vi "GEA3 Read Write Example.vi"() -> ()   [LabVIEW 2020]
uses:
  type defs/ERD Write Data In.ctl
  type defs/Data Type.ctl
  type defs/ERD Read Data Out.ctl
  type defs/Source_Destination.ctl
  type defs/ERD Read Data In.ctl
  library/GEA2_Toolkit.lvlib
panel:
  out "String":string
  in  "Personality":string(combo)
  out "ERD Read Data Out":T1 {"ERD Number" format="%.0x"}
  in  "ERD Write Data In":T2 {"ERD Number" format="%.0x"}
  out "Raw Data Out":string
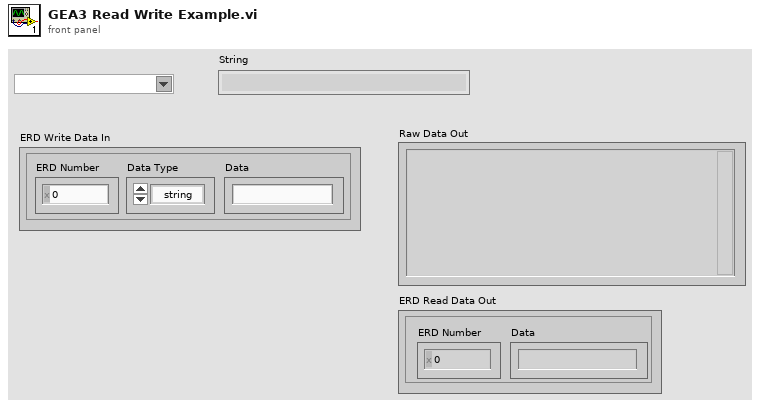
[diagram p1: front panel]
types:
  T1 = typedef "GEA2_Toolkit.lvlib/ERD Read Data Out.ctl" = cluster{"ERD Number":u16, "Data":string}
  T2 = typedef "GEA2_Toolkit.lvlib/ERD Write Data In.ctl" = cluster{"ERD Number":u16, "Data Type":T3, "Data":string}
  T3 = typedef "GEA2_Toolkit.lvlib/Data Type.ctl" = enum16{"string", "boolean", "uint8_t", "uint16_t", "uint32_t", "uint64_t", "int8_t", "int16_t", "int32_t", "int64_t"}
  T4 = typedef "GEA2_Toolkit.lvlib/ERD Read Data In.ctl" = cluster{"ERD Number":u16, "Data Type":T3}
  T5 = typedef "GEA2_Toolkit.lvlib/Source_Destination.ctl" = cluster{"Source":u8, "Destination":u8}
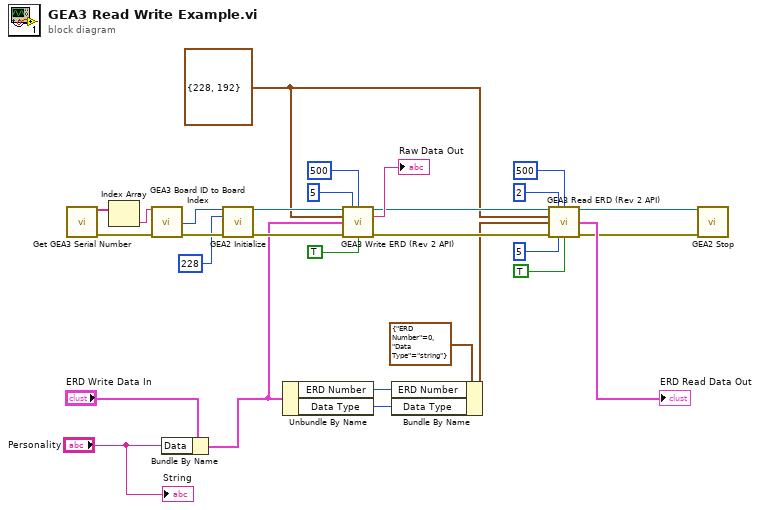
[diagram p0: block diagram]
diagram:
  w4 = T5 {"Source"=228, "Destination"=192} ("GEA Inputs")
  n1 = call "Get GEA3 Serial Number.vi"() -> ("GEA3 Serial Numbers"=w26:string[], "Error Out"=w27:errorcluster)  [unwired: 14 in]
  n2 = Index Array(array=w26) -> (element=w25:string)  [unwired: 1 in]
  n3 = call "GEA3 Board ID to Board Index.vi"("GEA3 Serial Number"=w25, "Error In"=w27) -> ("Board Index"=w28:i32, "Error Out"=w29:errorcluster)  [unwired: 9 in, 3 out]
  n4 = Bundle By Name(cluster="ERD Write Data In", "Data"="Personality") -> (w2:T2)
  n5 = call "GEA2 Initialize.vi"("Board Index"=w28, "Source Address"=u8 228, "error in"=w29) -> ("GEA2 Reference Out"=w23:refnum<k24>, "error out"=w24:errorcluster)  [unwired: 10 in, 1 out]
  n6 = Unbundle By Name(w2) -> ("ERD Number"=w16:u16, "Data Type"=w15:T3)
  n7 = call "GEA3 Write ERD (Rev 2 API).vi"("GEA2 Reference In"=w23, "# of Tries"=u8 5, "Read Timeout (ms)"=u32 500, "GEA Inputs"=w4, "ERD Write Data In"=w2, "Error In"=w24, "Verify ERD Response?"=TRUE) -> ("GEA2 Reference Out"=w18:refnum<k24>, "Raw Data Out"=→"Raw Data Out":string, "Error Out"=w19:errorcluster)  [unwired: 5 in, 1 out]
  n8 = Bundle By Name(cluster=T4 {"ERD Number"=0, "Data Type"=enum."string"} ("ERD Read Data In"), "ERD Number"=w16, "Data Type"=w15) -> (w14:T4)
  n9 = call "GEA3 Read ERD (Rev 2 API).vi"("GEA2 Reference In"=w18, "Retry Count"=2, "Read Timeout (ms)"=u32 500, "GEA Inputs"=w4, "ERD Read Data In"=w14, "Error In"=w19, "Low Level Tries"=u8 5, "Verify ERD Response?"=TRUE) -> ("GEA2 Reference Out"=w6:refnum<k24>, "ERD Read Data Out"=→"ERD Read Data Out":T1, "Error Out"=w5:errorcluster)  [unwired: 4 in, 1 out]
  n10 = call "GEA2 Stop.vi"("GEA2 Reference In"=w6, "Error In"=w5) -> ()  [unwired: 13 in, 1 out]
  "String" <- "Personality"
